vi "ProjetoOsciloscopio (1) (1).vi"() -> ()   [LabVIEW 2019]
uses:
  Control 1.ctl
panel:
  in  "Canais 1 e 2 - XY":bool
  out "XY Graph":cluster{"Y":dbl[], "Y":dbl[]}[](graph)
  in  "Phase 2":dbl caption="Phase"
  in  "Amplitude 2":dbl=1.0 caption="Amplitude"
  in  "Frequency 2":dbl=10.1 caption="Frequency"
  in  "Offset 2":dbl caption="Offset"
  out "error out":errorcluster
  in  "Phase 1":dbl caption="Phase"
  in  "Amplitude 1":dbl=2.0 caption="Amplitude"
  in  "Frequency 1":dbl=10.1 caption="Frequency"
  in  "Offset 1":dbl caption="Offset"
  in  "Operação":enum16{"Subtração", "Soma"}(ring)
  out "RMS 3":dbl
  out "Vpp 3":dbl
  out "RMS 2":dbl
  in  "Math":bool
  out "Vpp 2":dbl
  out "RMS 1":dbl
  out "Vpp 1":dbl
  in  "Canal 1":bool
  in  "Canal 2":bool
  out "error out 2":errorcluster caption="error out"
  out "Waveform Graph":T1
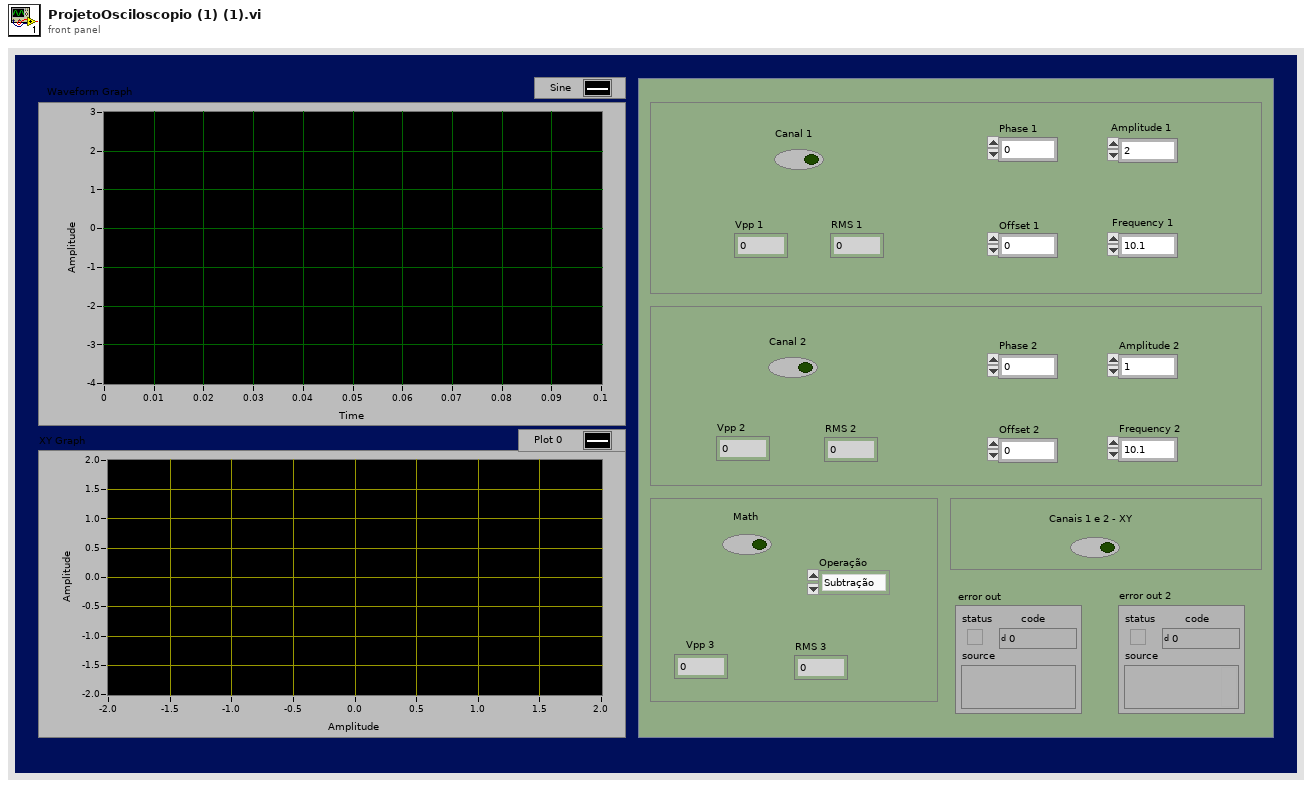
[diagram p1: front panel]
types:
  T1 = typedef "Control 1.ctl" = dynamicdata
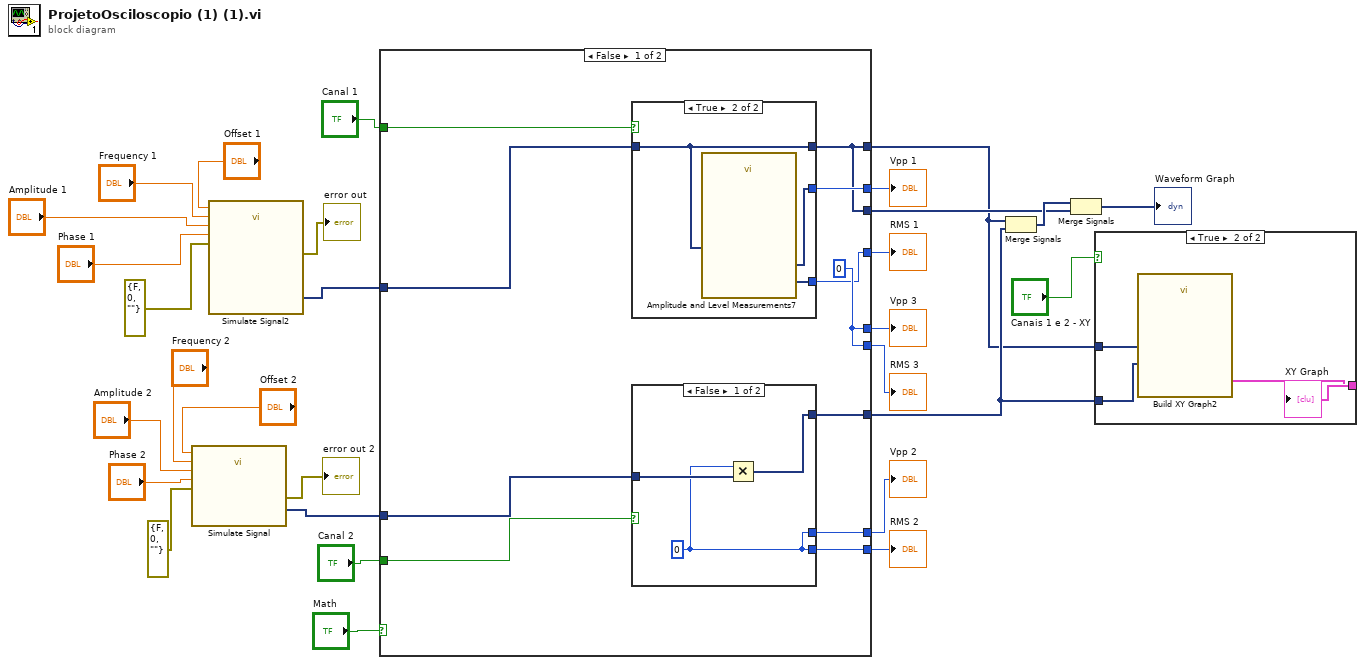
[diagram p0: block diagram]
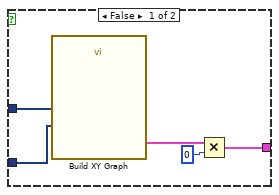
[diagram p2: hidden frame]
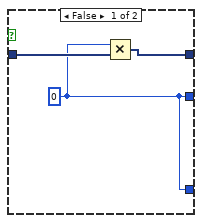
[diagram p3: hidden frame]
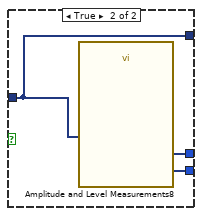
[diagram p4: hidden frame]
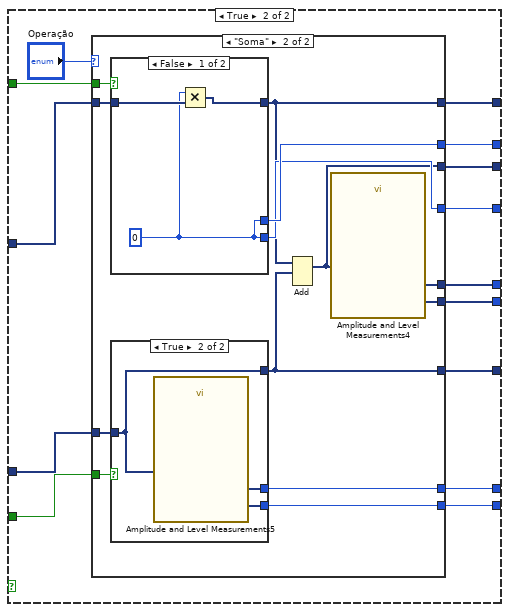
[diagram p5: hidden frame]
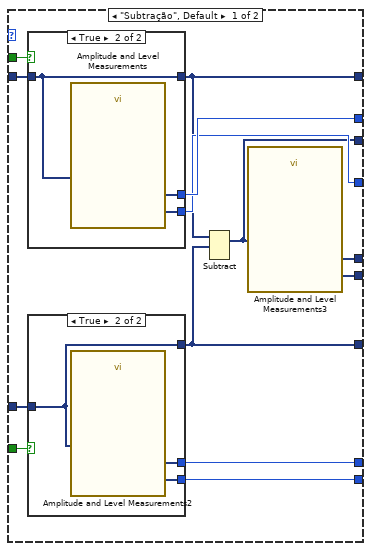
[diagram p6: hidden frame]
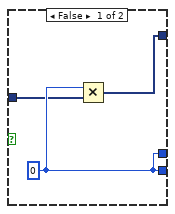
[diagram p7: hidden frame]
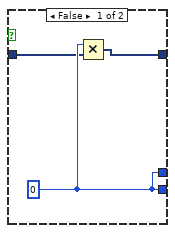
[diagram p8: hidden frame]
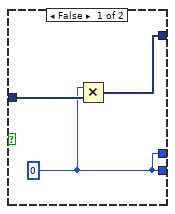
[diagram p9: hidden frame]
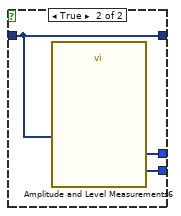
[diagram p10: hidden frame]
diagram:
  n1 = call "Simulate Signal"("Offset"="Offset 2", "Frequency"="Frequency 2", "Amplitude"="Amplitude 2", "Phase"="Phase 2", "error in (no error)"=errorcluster {"status"=FALSE, "code"=0, "source"=""}) -> ("Sine"=w1:dynamicdata, "error out"=→"error out 2":errorcluster)  [unwired: 9 in]
  n2 = call "Simulate Signal2"("Offset"="Offset 1", "Frequency"="Frequency 1", "Amplitude"="Amplitude 1", "Phase"="Phase 1", "error in (no error)"=errorcluster {"status"=FALSE, "code"=0, "source"=""}) -> ("Sine"=w2:dynamicdata, "error out"=→"error out":errorcluster)  [unwired: 9 in]
  n3 = case shown="False" "Math" {
    tunnel: [w41 w56] -> w30
    tunnel: [w41 w57] -> w29
    tunnel: [w40 w66] -> w27
    tunnel: [w39 w65] -> w26
    tunnel: [w37 w64] -> w25
    tunnel: [w38 w63] -> w24
    tunnel: "Canal 1" -> [w34 w62]
    tunnel: "Canal 2" -> [w35 w61]
    tunnel: [w36 w60] -> w4
    tunnel: [w31 w59] -> w3
    tunnel: [w31 w58] -> w5
    tunnel: w2 -> [w33 w55]
    tunnel: w1 -> [w32 w54]
    frame False {
      w41 = 0
      n4 = case shown="True" w34 {
        tunnel: [w43 w47] -> w40
        tunnel: [w43 w46] -> w39
        tunnel: [w42 w45] -> w31
        tunnel: w33 -> [w44 w45]
        frame False {
          w43 = 0
          n5 = Multiply(x=w43, y=w44) -> (x*y=w42:dynamicdata)
        }
        frame True {
          n6 = call "Amplitude and Level Measurements7"("Signals"=w45) -> ("RMS"=w46:dynamicdata, "Peak to Peak"=w47:dynamicdata)  [unwired: 12 in, 1 out]
        }
      }
      n7 = case shown="False" w35 {
        tunnel: [w48 w53] -> w38
        tunnel: [w48 w52] -> w37
        tunnel: [w50 w51] -> w36
        tunnel: w32 -> [w49 w51]
        frame False {
          w48 = 0
          n8 = Multiply(x=w48, y=w49) -> (x*y=w50:dynamicdata)
        }
        frame True {
          n9 = call "Amplitude and Level Measurements8"("Signals"=w51) -> ("RMS"=w52:dynamicdata, "Peak to Peak"=w53:dynamicdata)  [unwired: 12 in, 1 out]
        }
      }
    }
    frame True {
      n10 = case shown="\"Soma\"" "Operação" {
        tunnel: [w78 w105] -> w66
        tunnel: [w77 w104] -> w65
        tunnel: [w75 w100] -> w64
        tunnel: [w76 w101] -> w63
        tunnel: w62 -> [w80 w103]
        tunnel: w61 -> [w79 w102]
        tunnel: [w74 w98] -> w60
        tunnel: [w69 w99] -> w59
        tunnel: [w68 w97] -> w58
        tunnel: [w73 w95] -> w57
        tunnel: [w72 w96] -> w56
        tunnel: w55 -> [w71 w94]
        tunnel: w54 -> [w70 w93]
        frame "Subtração", Default {
          n11 = case shown="True" w80 {
            tunnel: [w89 w92] -> w78
            tunnel: [w89 w91] -> w77
            tunnel: w71 -> [w88 w90]
            tunnel: [w87 w90] -> w69
            frame False {
              w89 = 0
              n12 = Multiply(x=w89, y=w88) -> (x*y=w87:dynamicdata)
            }
            frame True {
              n13 = call "Amplitude and Level Measurements"("Signals"=w90) -> ("RMS"=w91:dynamicdata, "Peak to Peak"=w92:dynamicdata)  [unwired: 12 in, 1 out]
            }
          }
          n14 = case shown="True" w79 {
            tunnel: [w83 w86] -> w76
            tunnel: [w83 w85] -> w75
            tunnel: [w81 w84] -> w74
            tunnel: w70 -> [w82 w84]
            frame False {
              w83 = 0
              n15 = Multiply(x=w83, y=w82) -> (x*y=w81:dynamicdata)
            }
            frame True {
              n16 = call "Amplitude and Level Measurements2"("Signals"=w84) -> ("RMS"=w85:dynamicdata, "Peak to Peak"=w86:dynamicdata)  [unwired: 12 in, 1 out]
            }
          }
          n17 = Subtract(1:w74, 2:w69) -> (0:w68:dynamicdata)  [unwired: 1 in, 1 out]
          n18 = call "Amplitude and Level Measurements3"("Signals"=w68) -> ("RMS"=w72:dynamicdata, "Peak to Peak"=w73:dynamicdata)  [unwired: 12 in, 1 out]
        }
        frame "Soma" {
          n19 = case shown="False" w103 {
            tunnel: [w112 w117] -> w105
            tunnel: [w112 w116] -> w104
            tunnel: [w114 w115] -> w99
            tunnel: w94 -> [w113 w115]
            frame False {
              w112 = 0
              n20 = Multiply(x=w112, y=w113) -> (x*y=w114:dynamicdata)
            }
            frame True {
              n21 = call "Amplitude and Level Measurements6"("Signals"=w115) -> ("RMS"=w116:dynamicdata, "Peak to Peak"=w117:dynamicdata)  [unwired: 12 in, 1 out]
            }
          }
          n22 = case shown="True" w102 {
            tunnel: [w107 w111] -> w101
            tunnel: [w107 w110] -> w100
            tunnel: [w106 w109] -> w98
            tunnel: w93 -> [w108 w109]
            frame False {
              w107 = 0
              n23 = Multiply(x=w107, y=w108) -> (x*y=w106:dynamicdata)
            }
            frame True {
              n24 = call "Amplitude and Level Measurements5"("Signals"=w109) -> ("RMS"=w110:dynamicdata, "Peak to Peak"=w111:dynamicdata)  [unwired: 12 in, 1 out]
            }
          }
          n25 = Add(1:w98, 2:w99) -> (0:w97:dynamicdata)  [unwired: 1 in, 1 out]
          n26 = call "Amplitude and Level Measurements4"("Signals"=w97) -> ("RMS"=w96:dynamicdata, "Peak to Peak"=w95:dynamicdata)  [unwired: 12 in, 1 out]
        }
      }
    }
  }
  "RMS 3" <- w30
  "Vpp 3" <- w29
  "Vpp 1" <- w27
  "RMS 1" <- w26
  "RMS 2" <- w25
  "Vpp 2" <- w24
  n27 = Merge Signals(w3, w4) -> (w7:dynamicdata)
  n28 = Merge Signals(w7, w5) -> (→"Waveform Graph":dynamicdata)
  n29 = case shown="True" "Canais 1 e 2 - XY" {
    tunnel: [w118 w125] -> w9
    tunnel: w3 -> [w122 w124]
    tunnel: w4 -> [w121 w123]
    frame False {
      n30 = call "Build XY Graph"("Y Input"=w121, "X Input"=w122) -> ("XY Graph"=w119:cluster{"X":dbl[], "Y":dbl[]}[])  [unwired: 8 in, 1 out]
      n31 = Multiply(x=w119, y=0) -> (x*y=w118:cluster{"X":dbl[], "Y":dbl[]}[])
    }
    frame True {
      n32 = call "Build XY Graph2"("Y Input"=w123, "X Input"=w124) -> ("XY Graph"=w125:cluster{"X":dbl[], "Y":dbl[]}[])  [unwired: 8 in, 1 out]
    }
  }
  "XY Graph" <- w9
